vi "acquireConstantSamples.vi"(0 "Instrument handle":refnum<k15>, 1 "Channel(s)":string, 2 "Cycles to acquire":u16=1 min=1, 3 "Samples/cycle":u32=1000 min=1, 4 "Frequency":dbl min=0.0 step=1000.0 format="%#_6p", 5 "error in (no error)":errorcluster) -> (13 "Waveform(s)":waveform(dbl)[](graph), 14 "Instrument handle out":refnum<k15>, 15 "Requested record length":i32, 16 "Reqested sample rate":dbl, 17 "Actual record length":i32=1000, 18 "Actual sample rate":dbl=10000000.0 format="%#.2p", 19 "error out":errorcluster)   [LabVIEW 2020]
uses:
  <instrlib>/niScope/Acquire/Fetch/niScope Multi Fetch WDT.vi
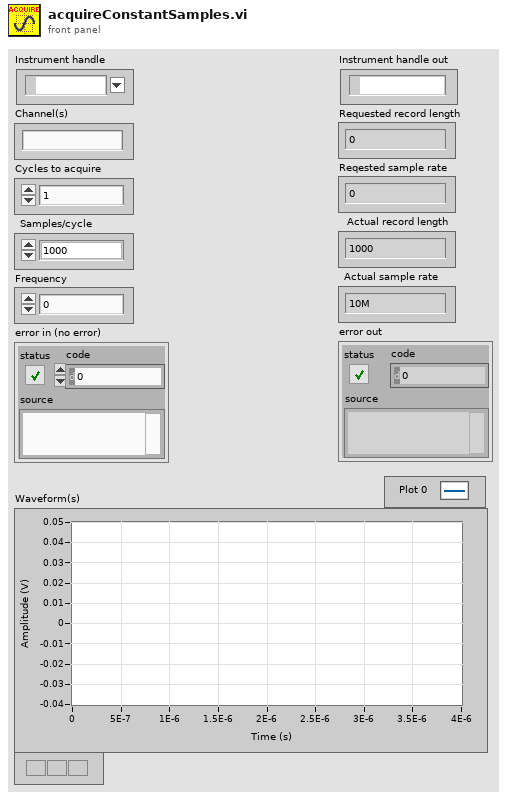
[diagram p1: front panel]
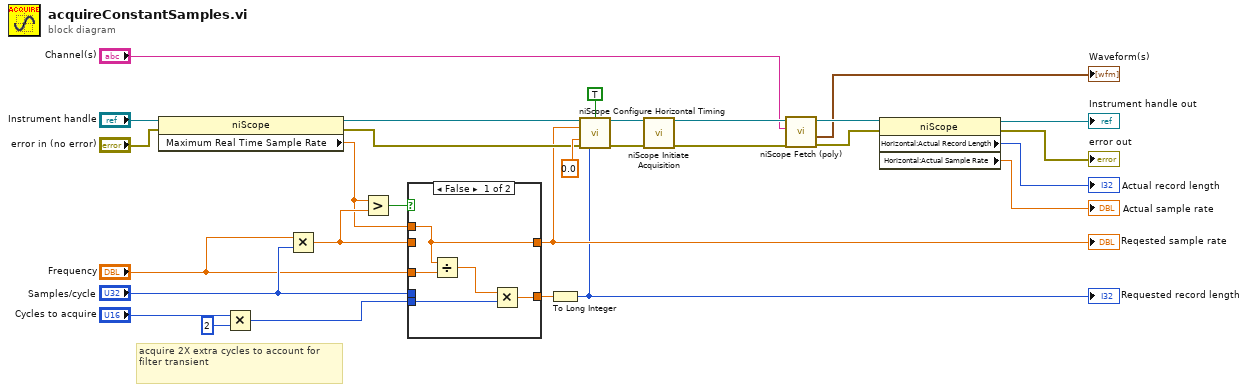
[diagram p0: block diagram]
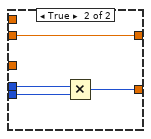
[diagram p2: hidden frame]
diagram:
  # "acquire 2X extra cycles to account for filter transient"
  n1 = property class="niScope"(reference="Instrument handle", error in="error in (no error)") -> (reference out=w14:refnum<k15>, error out=w13:errorcluster, "Maximum Real Time Sample Rate"=w6:dbl)
  n2 = Multiply(x="Cycles to acquire", y=u16 2) -> (x*y=w1:u16)
  n3 = Multiply(x="Frequency", y="Samples/cycle") -> (x*y=w8:dbl)
  n4 = Greater?(x=w6, y=w8) -> (0:w10:bool)
  n5 = case shown="False" w10 {
    tunnel: w1 -> [w30 w38]
    tunnel: "Samples/cycle" -> [_ w37]
    tunnel: [w32 w36] -> w5
    tunnel: "Frequency" -> [w34 _]
    tunnel: w8 -> [_ w35]
    tunnel: [w33 w35] -> w7
    tunnel: w6 -> [w33 _]
    frame False {
      n6 = Divide(x=w33, y=w34) -> (x/y=w31:dbl)
      n7 = Multiply(x=w31, y=w30) -> (x*y=w32:dbl)
    }
    frame True {
      n8 = Multiply(x=w37, y=w38) -> (x*y=w36:u32)
    }
  }
  "Reqested sample rate" <- w7
  n9 = To Long Integer(number=w5) -> (32bit integer=w4:i32)
  "Requested record length" <- w4
  n10 = call <instrlib>:"niScope Configure Horizontal Timing.vi"("instrument handle"=w14, "enforce realtime"=TRUE, "min sample rate"=w7, "reference position"=0.0, "error in"=w13, "min record length"=w4) -> ("instrument handle out"=w27:refnum<k15>, "error out"=w26:errorcluster)  [unwired: 8 in]
  n11 = call <instrlib>:"niScope Initiate Acquisition.vi"("instrument handle"=w27, "error in"=w26) -> ("instrument handle out"=w25:refnum<k15>, "error out"=w24:errorcluster)  [unwired: 12 in]
  n12 = call-poly <instrlib>:"niScope Fetch (poly).vi"("error in"=w24, "channels"="Channel(s)", "instrument handle"=w25) -> ("error out"=w17:errorcluster, "wfm"=→"Waveform(s)":waveform(dbl)[], "instrument handle out"=w29:refnum<k15>)  [unwired: 5 in, 1 out]
  n13 = property class="niScope"(reference=w29, error in=w17) -> (reference out=→"Instrument handle out":refnum<k15>, error out=→"error out":errorcluster, "Horizontal:Actual Record Length"=→"Actual record length":i32, "Horizontal:Actual Sample Rate"=→"Actual sample rate":dbl)
